vi "lockin - add phase element.vi"(8 "error in (no error)":errorcluster, 11 "Lockin":refnum<class "Instrument.Lockin.lvclass">) -> (0 "error out":errorcluster, 3 "Lockin out":refnum<class "Instrument.Lockin.lvclass">)   [LabVIEW 2016, in "Instrument.Lockin.lvclass"]
uses:
  Instrument.Lockin.lvclass
  Instrument.Lockin.lvclass/Instrument.Lockin.ctl
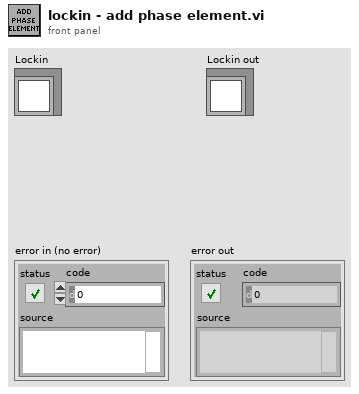
[diagram p1: front panel]
types:
  T1 = typedef "Instrument.Lockin.lvclass/REF-cluster.ctl" = cluster{"REF f (Hz)":T2, "REF phi (°)":T3}
  T2 = typedef "Instrument.Lockin.lvclass/REF_f-array.ctl" = dbl[]
  T3 = typedef "Instrument.Lockin.lvclass/REF_phi-array.ctl" = dbl[]
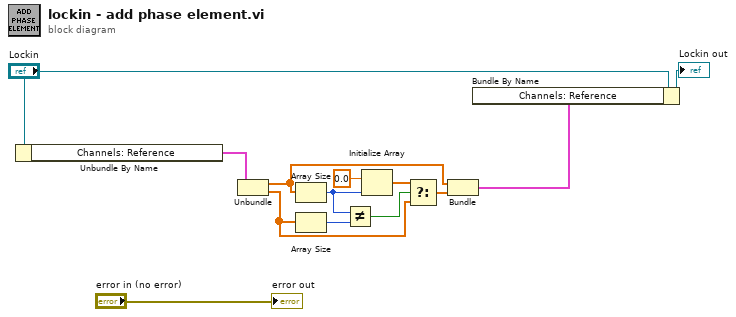
[diagram p0: block diagram]
diagram:
  n1 = Unbundle By Name("Lockin") -> ("Channels: Reference"=w5:T1)
  n2 = Unbundle(w5) -> ("REF f (Hz)"=w11:T2, "REF phi (°)"=w9:T3)
  n3 = Array Size(array=w11) -> (size(s)=w6:i32)
  n4 = Array Size(array=w9) -> (size(s)=w12:i32)
  n5 = Not Equal?(x=w6, y=w12) -> (x != y?=w13:bool)
  n6 = Initialize Array(0.0 ("element"), w6) -> (w8:dbl[])
  n7 = Select(t=w8, s=w13, f=w9) -> (s? t:f=w10:T3)
  n8 = Bundle("REF f (Hz)"=w11, "REF phi (°)"=w10) -> (w2:cluster{"REF f (Hz)":T2, "REF phi (°)":T3})  [unwired: 1 in]
  n9 = Bundle By Name(cluster="Lockin", "Channels: Reference"=w2) -> (→"Lockin out":refnum<class "Instrument.Lockin.lvclass">)
  "error out" <- "error in (no error)"
